vi "HexToFloat.vi"(11 "数组":u16[](array[numeric]) format="%04xH") -> (3 "FLOAT":sgl[](array[numeric]))   [LabVIEW 2016, in "氨氮总磷.lvlib"]
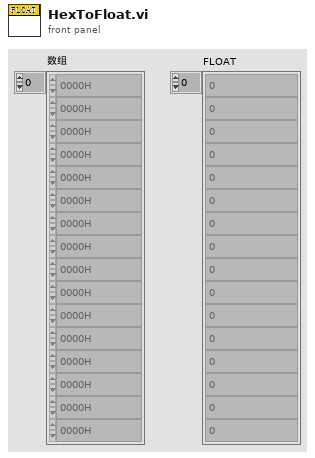
[diagram p1: front panel]
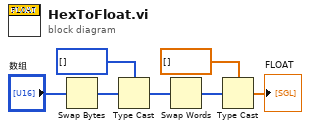
[diagram p0: block diagram]
diagram:
  n1 = Swap Bytes(anything="数组") -> (byte swapped=w5:u16[])
  n2 = Type Cast(type=u32[] [], x=w5) -> (*(type *) &x=w2:u32[])
  n3 = Swap Words(1:w2) -> (0:w1:u32[])
  n4 = Type Cast(type=sgl[] [], x=w1) -> (*(type *) &x=→"FLOAT":sgl[])
